vi "ClassAppData.Get All.vi"(8 "error in (no error)":errorcluster, 11 "Class - App Data in":refnum<class "Class.AppData.lvclass">) -> (0 "error out":errorcluster, 1 "Data Out":variant, 3 "Class - App Data out":refnum<class "Class.AppData.lvclass">)   [LabVIEW 2024, in "EQMF.lvlib" / "Config Utils.lvlib" / "Class.AppData.lvclass"]
doc: "<B>AppData Class:</B>\nThe AppData class keeps track of a library of data items that are used by an application. These data items have a name (text string) and value that can be any data type. \n\n<B>AppData.Get All VI:</B>\nThis VI outputs a variant that has all data dictionary items as attributes."
uses:
  Class.AppData.lvclass
  Class.AppData.lvclass/Class.AppData.ctl
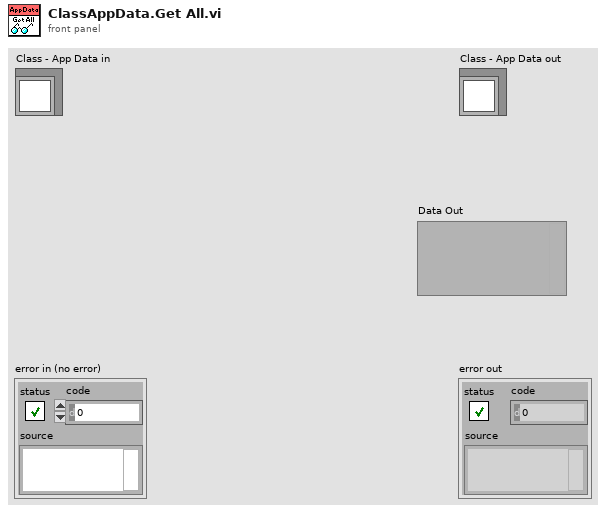
[diagram p1: front panel]
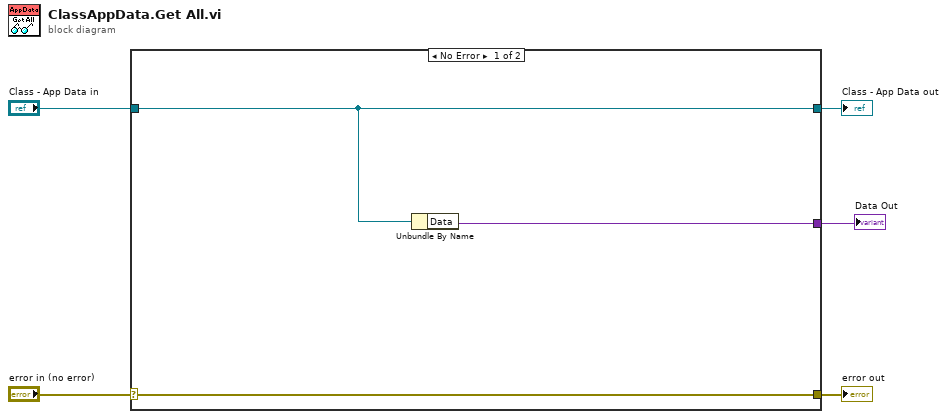
[diagram p0: block diagram]
diagram:
  n1 = case shown="No Error" "error in (no error)" {
    selector: "error in (no error)" -> [w6 w10]
    tunnel: [w6 w10] -> w4
    tunnel: [w8 w9] -> w2
    tunnel: "Class - App Data in" -> [w8 w9]
    tunnel: [w7 _] -> w1
    frame No Error {
      n2 = Unbundle By Name(w8) -> ("Data"=w7:variant)
    }
    frame Error {
    }
  }
  "error out" <- w4
  "Class - App Data out" <- w2
  "Data Out" <- w1
